vi "Teardown.vi"(8 "error in (no error)":errorcluster, 11 "LUnit Process Test In":refnum<class "Process Test.lvclass">) -> (0 "error out":errorcluster, 3 "LUnit Process Test Out":refnum<class "Process Test.lvclass">)   [LabVIEW 2020, in "Process Test.lvclass"]
uses:
  Process Test.lvclass
  Process Test.lvclass/Process Test.ctl
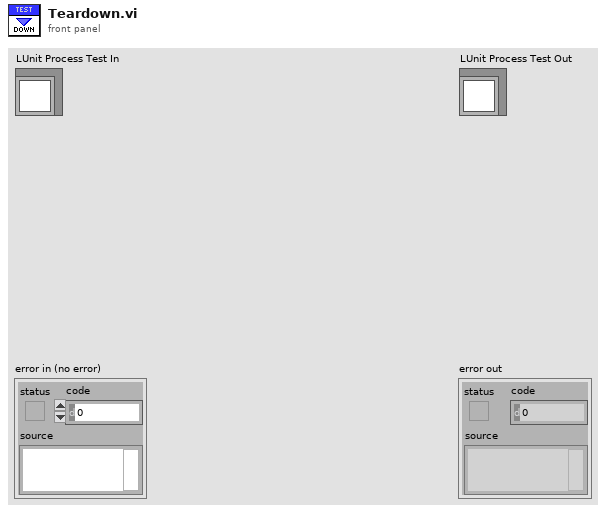
[diagram p1: front panel]
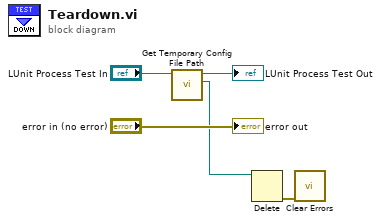
[diagram p0: block diagram]
diagram:
  n1 = call "Get Temporary Config File Path.vi"("Base Test in"="LUnit Process Test In") -> ("Temporary Config File Path"=w1:path, "Base Test out"=→"LUnit Process Test Out":refnum<class "Process Test.lvclass">)  [unwired: 8 in, 1 out]
  n2 = Delete(path (use dialog)=w1) -> (error out=w5:errorcluster)  [unwired: 4 in, 2 out]
  n3 = call <vilib>:"Clear Errors.vi"("error in (no error)"=w5) -> ()  [unwired: 5 in, 2 out]
  "error out" <- "error in (no error)"
